vi "Get ICommunicate.vi"(11 "DBC Communication in":refnum<class "DBC Communication.lvclass">) -> (2 "ICommunicate":refnum<class "ICommunicate.lvclass">, 3 "DBC Communication out":refnum<class "DBC Communication.lvclass">)   [LabVIEW 2024, in "DBC Communication.lvclass"]
uses:
  DBC Communication.lvclass
  Interfaces/ICommunicate/ICommunicate.lvclass
  DBC Communication.lvclass/DBC Communication.ctl
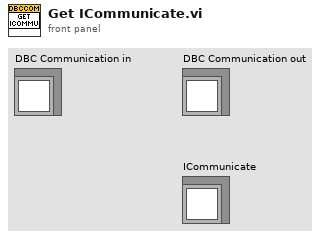
[diagram p1: front panel]
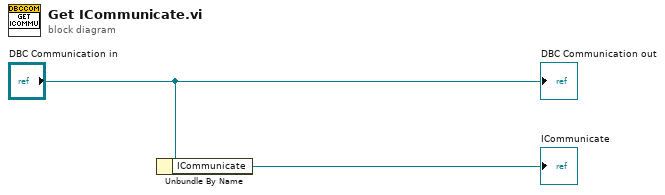
[diagram p0: block diagram]
diagram:
  n1 = Unbundle By Name("DBC Communication in") -> ("ICommunicate"=→"ICommunicate":refnum<class "ICommunicate.lvclass">)
  "DBC Communication out" <- "DBC Communication in"
